vi "INSPECT_Start Collect Helper.vi"(7 "Encoder Cnt":i32, 8 "error in (no error)":errorcluster, 9 "MaxSamples":i32, 10 "PosToEndScan":i32, 11 "EventLog in":refnum<class "EventLog.lvclass">) -> (0 "error out":errorcluster, 1 "Success":bool, 2 "data value reference":refnum<data-value>, 3 "Block Cnt notifier out":refnum<notifier>)   [LabVIEW 2015, in "Tool Module.lvlib"]
uses:
  Tool Module.lvlib
  Event Logger Library/Event Log/EventLog.lvclass
  Collect Data Mgr/Data Collect Parameters typedef--cluster.ctl
  Tool Interface/_HS Data Stream Params Cluster--typedef.ctl
  Collect Data Mgr/Start Collect (Reply Payload)--cluster.ctl
  ToolModGLOB.vi
  Tool Config/Tool Cfg.lvlib
  Collect Data Mgr/Collect Data Mgr.lvlib
  Tool Interface/Tool Interface.lvlib
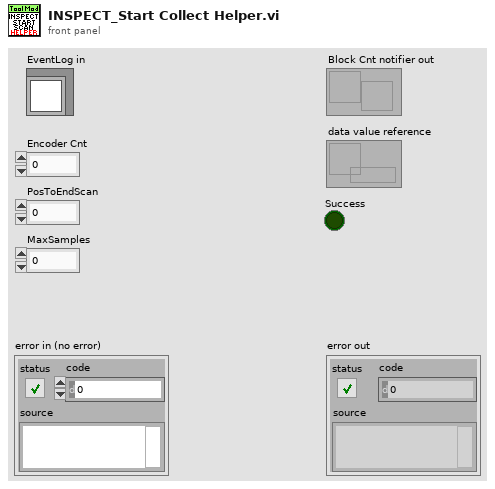
[diagram p1: front panel]
types:
  T1 = typedef "Collect Data Mgr.lvlib/Start Collect (Reply Payload)--cluster.ctl" = cluster{"Success":bool, "CD_Status":u8}
  T2 = enum16{"Idle", "Receive HS Data", "Close Connection"}
  T3 = typedef "Tool Interface.lvlib/_HS Data Stream Params Cluster--typedef.ctl" = cluster{"Raw Data Stream Loop cmd":enum16{"Idle", "Receive HS Data", "Close Connection"}, "Data Array DVR ref":refnum<data-value>, "Sample Data notifier":refnum<notifier>, "Block Count Notifier":refnum<notifier>}
  T4 = typedef "Collect Data Mgr.lvlib/Data Collect Parameters typedef--cluster.ctl" = cluster{"Mode":i8, "Move Length":i32, "Array Length":i32, "Max Samples":i32}
  T5 = typedef "Tool Cfg.lvlib/_Tool Operation Config Cluster--typedef.ctl" = cluster{"Use Tool Cfg":bool, "Use Tool Cal":bool, "Fake Data?":bool, "Mode":i16, "Array Subset Length":i16, "nArrays to Read":i16, "Full Array Read Length":i16, "nSubarrays/Sensor":i16}
  T6 = typedef "_Data Stream Fmt Params Cluster--typedef.ctl" = cluster{"Samples per Block":i32, "Raw Data Status Len":i32, "Fltr Data Status Len":i32}
  T7 = typedef "Tool Interface.lvlib/_Loop Ctrl Notifiers Cluster--typedef.ctl" = cluster{"Raw Stream Ctrl":refnum<notifier>}
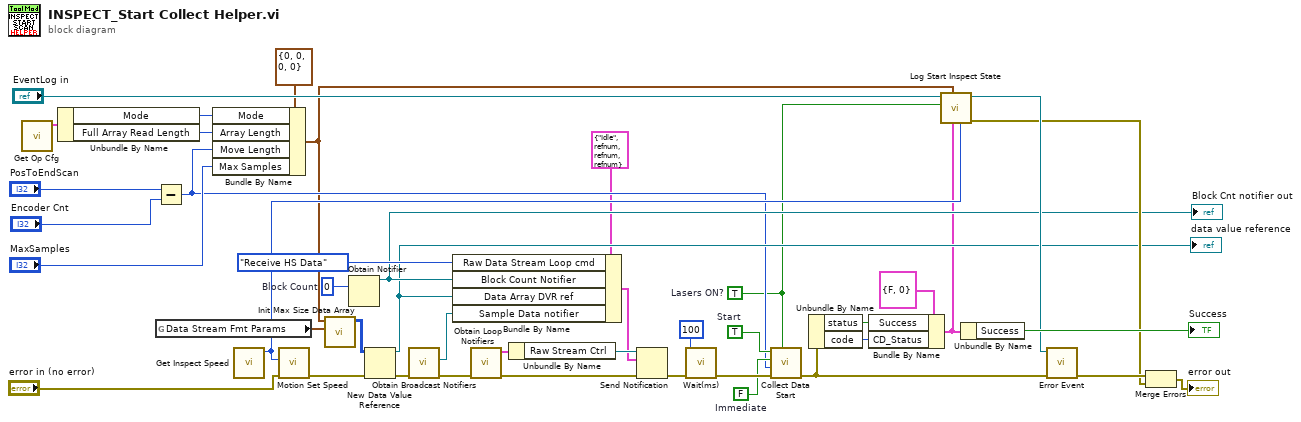
[diagram p0: block diagram]
diagram:
  w11 = FALSE  # Immediate
  w10 = TRUE  # Start
  w20 = u32 0  # Block Count
  w3 = TRUE  # Lasers ON?
  n1 = call "Get Op Cfg.vi"() -> ("Tool Operation Config"=w38:T5)  [unwired: 11 in]
  n2 = Unbundle By Name(w38) -> ("Mode"=w37:i16, "Full Array Read Length"=w36:i16)
  n3 = Subtract(x="PosToEndScan", y="Encoder Cnt") -> (x-y=w9:i32)
  n4 = global read "ToolModGLOB.vi" "Data Stream Fmt Params"() -> (w32:T6)
  n5 = Bundle By Name(cluster=T4 {"Mode"=0, "Move Length"=0, "Array Length"=0, "Max Samples"=0} ("_Data Collect Params typedef--cluster"), "Mode"=w37, "Array Length"=w36, "Move Length"=w9, "Max Samples"="MaxSamples") -> (w2:T4)
  n6 = call "Get Inspect Speed.vi"() -> ("Inspect Speed"=w39:u16)  [unwired: 11 in]
  n7 = call "Motion Set Speed.vi"("error in (no error)"="error in (no error)", "Speed"=w39) -> ("error out"=w30:errorcluster)  [unwired: 9 in]
  n8 = call "Init Max Size Data Array.vi"("Data Stream Fmt Params"=w32, "Data Collect Params"=w2) -> ("initialized array"=w31:u32[][])  [unwired: 9 in]
  n9 = Obtain Notifier(notification data type=w20) -> (notifier out=w19:refnum<notifier>)  [unwired: 3 in, 2 out]
  "Block Cnt notifier out" <- w19
  n10 = New Data Value Reference(data value=w31, error in=w30) -> (data value reference=w15:refnum<data-value>, error out=w18:errorcluster)
  "data value reference" <- w15
  n11 = call "Obtain Broadcast Notifiers.vi"("error in (no error)"=w18) -> ("Sample Data notifier out"=w14:refnum<notifier>)  [unwired: 9 in, 1 out]
  n12 = Bundle By Name(cluster=T3 {"Raw Data Stream Loop cmd"=enum."Idle", "Data Array DVR ref"=refnum, "Sample Data notifier"=refnum, "Block Count Notifier"=refnum} ("Cluster"), "Raw Data Stream Loop cmd"=T2."Receive HS Data" ("HS Data Stream SM enum"), "Block Count Notifier"=w19, "Data Array DVR ref"=w15, "Sample Data notifier"=w14) -> (w16:T3)
  n13 = call "Obtain Loop Notifiers.vi"("error in (no error)"=w18) -> ("error out"=w17:errorcluster, "Loop Ctrl Notifiers Cluster"=w22:T7)  [unwired: 9 in]
  n14 = Unbundle By Name(w22) -> ("Raw Stream Ctrl"=w21:refnum<notifier>)
  n15 = Send Notification(notification=w16, notifier=w21, error in (no error)=w17) -> (error out=w12:errorcluster)  [unwired: 1 out]
  n16 = call "Wait(ms).vi"("error in (no error)"=w12, "milliseconds"=u32 100) -> ("error out"=w41:errorcluster)  [unwired: 9 in]
  n17 = call "Collect Data Start.vi"("Lasers ON?"=w3, "error in (no error)"=w41, "Length"=w9, "Immediate"=w11, "Start"=w10) -> ("error out"=w4:errorcluster)  [unwired: 6 in]
  n18 = Unbundle By Name(w4) -> ("status"=w8:bool, "code"=w6:i32)
  n19 = Bundle By Name(cluster=T1 {"Success"=FALSE, "CD_Status"=0} ("Start Collect (Reply Payload)"), "Success"=w8, "CD_Status"=w6) -> (w5:T1)
  n20 = call "Log Start Inspect State.vi"("Speed"=w39, "Start Collect (Reply Payload)"=w5, "Data Collect Params"=w2, "Laser On"=w3, "EventLog in"="EventLog in") -> ("error out"=w24:errorcluster, "EventLog out"=w28:refnum<class "EventLog.lvclass">)  [unwired: 5 in]
  n21 = Unbundle By Name(w5) -> ("Success"=→"Success":bool)
  n22 = call "Error Event.vi"("error in (no error)"=w4, "EventLog ref"=w28) -> ("error out"=w25:errorcluster)  [unwired: 8 in, 1 out]
  n23 = Merge Errors(w25, w24) -> (→"error out":errorcluster)
